vi "Handle Inlet Return.vi"(8 "error in":errorcluster, 11 "Log Session":T1) -> (0 "error out":errorcluster, 2 "Filter State":bool, 3 "Log Session Out":T1)   [LabVIEW 2014, in "Controller.lvlib" / "Controller.lvclass"]
uses:
  Controller.lvclass
  <userlib>/_Session Fwk/Typedefs/Session Handle.ctl
  <userlib>/_Session Fwk/Session - Root.lvclass
  <vilib>/DAQmx/read.llb/DAQmx Read (Digital 1D Bool NChan 1Samp 1Line).vi
  <vilib>/DAQmx/write.llb/DAQmx Write (Digital Bool 1Line 1Point).vi
  reusable/Session APIs/Session Log/System Log.lvclass
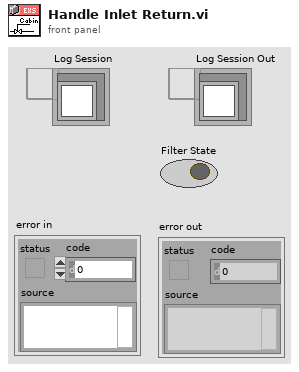
[diagram p1: front panel]
types:
  T1 = typedef "Session - Root.lvclass/Session Handle.ctl" = refnum<data-value>
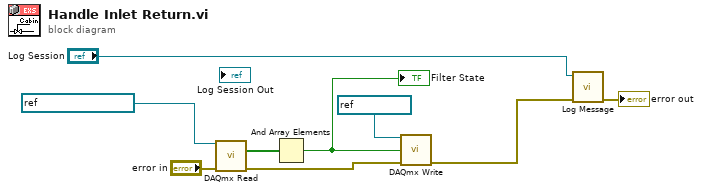
[diagram p0: block diagram]
diagram:
  n1 = call-poly <vilib>:"DAQmx Read.vi"("task/channels in"=refnum<k21> "Cabn Valve RTN", "error in"="error in") -> ("data"=w8:bool[], "error out"=w7:errorcluster)  [unwired: 11 in, 1 out]
  n2 = And Array Elements(Boolean array=w8) -> (logical AND=w9:bool)
  "Filter State" <- w9
  n3 = call-poly <vilib>:"DAQmx Write.vi"("task/channels in"=refnum<k21> "Inlet LED", "data"=w9, "error in"=w7) -> ("error out"=w5:errorcluster)  [unwired: 10 in, 2 out]
  n4 = call "Log Message.vi"("error in"=w5, "session in"="Log Session") -> ("error out"=→"error out":errorcluster)  [unwired: 8 in, 1 out]
